vi "Write Port.vi"(8 "error in (no error)":errorcluster, 9 "Port Mask":u64, 11 "Connection Data In":T1) -> (0 "error out":errorcluster, 3 "Connection Data Out":T1)   [LabVIEW 2014, in "MSX-E3701_dll.lvlib"]
doc: "Toma los datos enmascarados, hace un corrimiento y la dll se encarga de escribir las salidas digitales en función de la masca que se le paso (Port Mask)."
uses:
  MSX-E3701_dll.lvlib
  Typedef/Connection Data.ctl
  E:/Repositorio Magnis/INF002/v0/Modules/HAL/Drivers/Sync/ADDI-DATA MSX-E3701/API/MX370x.dll
  MX370x.dll
  E:/Repositorio Magnis/INF002/v0/Modules/HAL/Drivers/Sync/ADDI-DATA MSX-E3701/API/MXCommon.dll
  MXCommon.dll
panel:
  out "ESTATUS DE STOP DEL SISTEMA":string="Success"
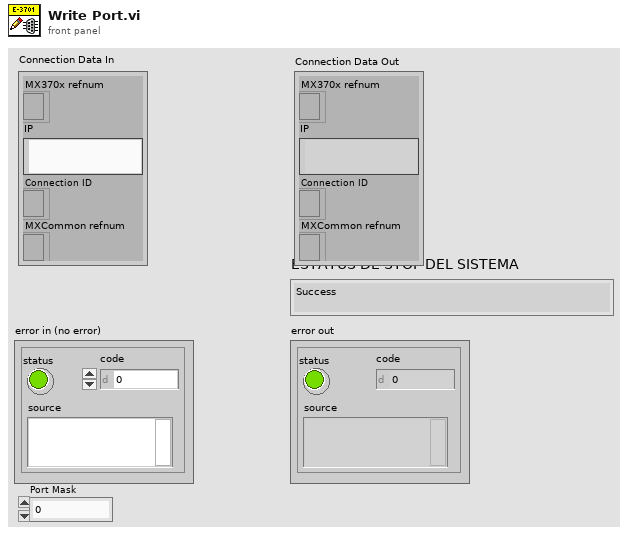
[diagram p1: front panel]
types:
  T1 = typedef "MSX-E3701_dll.lvlib/Connection Data.ctl" = cluster{"MX370x refnum":refnum<k24>, "IP":string, "Connection ID ":refnum<k5>, "MXCommon refnum":refnum<k24>}
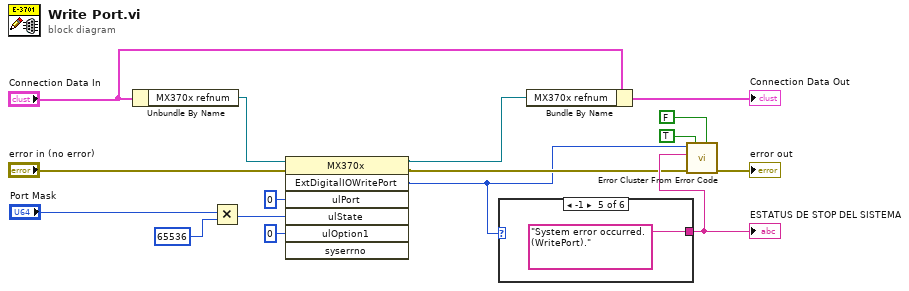
[diagram p0: block diagram]
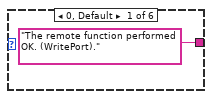
[diagram p2: hidden frame]
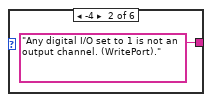
[diagram p3: hidden frame]
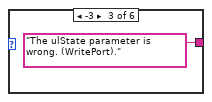
[diagram p4: hidden frame]
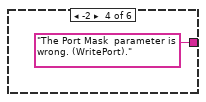
[diagram p5: hidden frame]
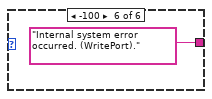
[diagram p6: hidden frame]
diagram:
  n1 = Unbundle By Name("Connection Data In") -> ("MX370x refnum"=w10:refnum<k24>)
  n2 = Multiply(x="Port Mask", y=u64 65536) -> (x*y=w2:u64)
  n3 = invoke class="MX370x" method="ExtDigitalIOWritePort"(reference=w10, error in="error in (no error)", "ulPort"=u64 0, "ulState"=w2, "ulOption1"=u64 0) -> (reference out=w8:refnum<k24>, error out=w7:errorcluster, "ExtDigitalIOWritePort"=w6:i32)  [unwired: 2 in, 4 out]
  n4 = case shown="-1" w6 {
    tunnel: ["The remote function performed OK. (WritePort)." "Any digital I/O set to 1 is not an output channel. (WritePort)." "The ulState parameter is wrong. (WritePort)." "The Port Mask  parameter is wrong. (WritePort)." "System error occurred. (WritePort)." "Internal system error occurred. (WritePort)."] -> w13
    frame 0, Default {
    }
    frame -4 {
    }
    frame -3 {
    }
    frame -2 {
    }
    frame -1 {
    }
    frame -100 {
    }
  }
  "ESTATUS DE STOP DEL SISTEMA" <- w13
  n5 = Bundle By Name(cluster="Connection Data In", "MX370x refnum"=w8) -> (→"Connection Data Out":T1)
  n6 = call <vilib>:"Error Cluster From Error Code.vi"("is warning? (False)"=FALSE, "show call chain? (False)"=TRUE, "error in (no error)"=w7, "error message (\"\")"=w13, "error code (0)"=w6) -> ("error out"=→"error out":errorcluster)  [unwired: 4 in]
